vi "TEST_LoadSpec.vi"(7 "Drain!Fill":bool=TRUE, 9 "Index":i32, 10 "Level IN inches":dbl=5.0, 11 "Full Cfg in":T3={"Bench Config"={"Name"="OLR001", {"Step Levels"=0.05, "Tolerance"=0.01, "Sample Rate"=0.05, "Resistor"=100.0, "M Level Cal"=1.0, "[B Level Cal"=0.0, "Max Fill Rate"=0.002, "Empty Inches"=8.0, "Full Inches"=2.6}}, "Test Value Table "=[[98.0, 102.0, 8.5, 8.5, 8.5, 8.5, 98.0, 102.0, 8.5, 8.5, 8.5, 8.5], [98.0, 102.0, 7.91, 8.01, 7.55, 7.65, 98.0, 102.0, 7.685, 7.785, 7.325, 7.425], [197.0, 203.0, 7.46, 7.56, 7.1, 7.2, 197.0, 203.0, 7.235, 7.335, 6.875, 6.975], [296.0, 304.0, 7.01, 7.11, 6.65, 6.75, 296.0, 304.0, 6.785, 6.885, 6.425, 6.525], [395.0, 405.0, 6.56, 6.66, 6.2, 6.3, 395.0, 405.0, 6.335, 6.435, 5.975, 6.075], [494.0, 506.0, 6.11, 6.21, 5.75, 5.85, 494.0, 506.0, 5.885, 5.985, 5.525, 5.625], [593.0, 607.0, 5.66, 5.76, 5.3, 5.4, 593.0, 607.0, 5.435, 5.535, 5.075, 5.175], [692.0, 708.0, 5.21, 5.31, 4.85, 4.95, 692.0, 708.0, 4.985, 5.085, 4.625, 4.725], [791.0, 809.0, 4.76, 4.86, 4.4, 4.5, 791.0, 809.0, 4.535, 4.635, 4.175, 4.275], [890.0, 910.0, 4.31, 4.41, 3.95, 4.05, 890.0, 910.0, 4.085, 4.185, 3.725, 3.825], [989.0, 1011.0, 3.86, 3.96, 3.5, 3.6, 989.0, 1011.0, 3.635, 3.735, 3.275, 3.375], [1088.0, 1112.0, 3.41, 3.51, 3.05, 3.15, 1088.0, 1112.0, 3.185, 3.285, 2.825, 2.925], [1088.0, 1112.0, 2.5, 2.5, 2.5, 2.5, 1088.0, 1112.0, 2.5, 2.5, 2.5, 2.5]], "Table Col Titles"=[["Aohm Lo", "Aohm Hi", "A Fill Lo", "A Fill Hi", "A Drain Lo", "A Drain Hi", "Bohm Lo", "Bohm Hi", "B Fill Lo", "B Fill Hi", "B Drain Lo", "B Drain Hi"]], "cluster"={"Fill "=refnum, "Drain"=refnum, "Level PV"=refnum, "Pump Speed"=refnum, "Run Test"=refnum, "Sim"=refnum, "Jog"=refnum, "Level SP"=refnum}, "Bench Status"={"Pump Status"=refnum, "Instrumnet\n Status"=refnum}}) -> (2 "Set Point":dbl=8.5, 3 "Array":T1[](array[typedef])=[{"Specs"=[8.5, 8.5, 0.0, 102.0, 98.0, 0.0, 0.0], "LUT Status"={"ChA/!ChB"=TRUE, "Drain/!Fill"=FALSE, "In Range?"=FALSE, "Switch Range?"=FALSE, "Measure R?"=FALSE, "Vaild R?"=FALSE, "Index(n)"=0, "Index(n)-1"=0, "Index Max"=13, "Index(n-1)"=-1}}, {"Specs"=[0.0, 0.0, 0.0, 0.0, 0.0, 0.0, 0.0], "LUT Status"={"ChA/!ChB"=FALSE, "Drain/!Fill"=FALSE, "In Range?"=FALSE, "Switch Range?"=FALSE, "Measure R?"=FALSE, "Vaild R?"=FALSE, "Index(n)"=-1, "Index(n)-1"=0, "Index Max"=13, "Index(n-1)"=-2}}])   [LabVIEW 2024]
uses:
  Control Definitions/Def FullCfg.ctl
  Control Definitions/Def BenchCfg.ctl
  Control Definitions/Def PumpCtlRefs.ctl
  Control Definitions/Def_PumpSpeed.ctl
  Control Definitions/Def Bench Status.ctl
  Control Definitions/Def Spec RNG.ctl
  Control Definitions/Ded LUT_Status.ctl
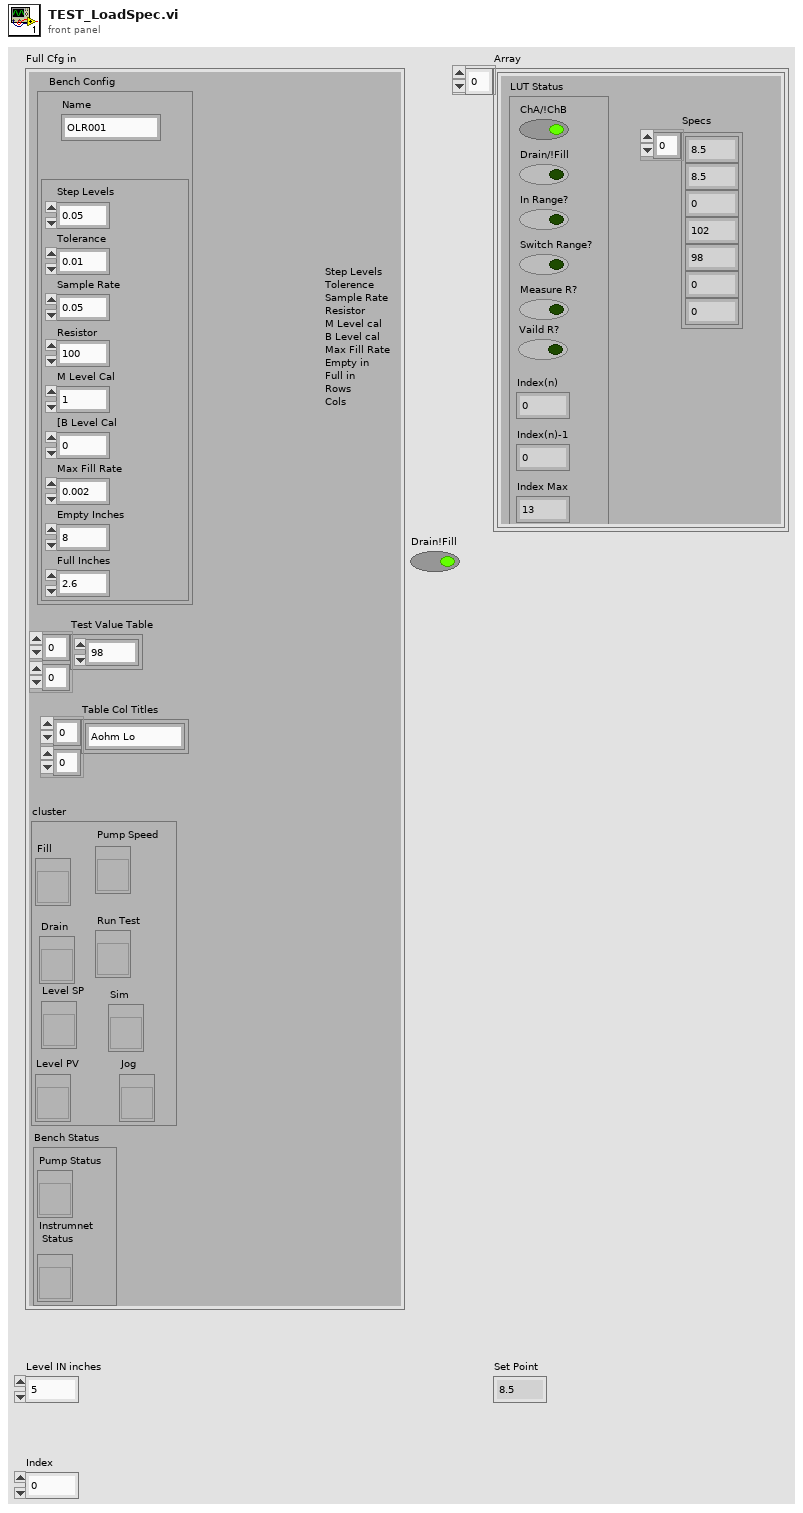
[diagram p1: front panel]
types:
  T1 = typedef "Def Spec RNG.ctl" = cluster{"Specs":dbl[], "LUT Status":T2}
  T2 = typedef "Ded LUT_Status.ctl" = cluster{"ChA/!ChB":bool, "Drain/!Fill":bool, "In Range?":bool, "Switch Range?":bool, "Measure R?":bool, "Vaild R?":bool, "Index(n)":i32, "Index(n)-1":i32, "Index Max":i32, "Index(n-1)":i32}
  T3 = typedef "Def FullCfg.ctl" = cluster{"Bench Config":T4, "Test Value Table ":dbl[][], "Table Col Titles":string[][], "cluster":T5, "Bench Status":T6}
  T4 = typedef "Def BenchCfg.ctl" = cluster{"Name":string, cluster{"Step Levels":dbl, "Tolerance":dbl, "Sample Rate":dbl, "Resistor":dbl, "M Level Cal":dbl, "[B Level Cal":dbl, "Max Fill Rate":dbl, "Empty Inches":dbl, "Full Inches":dbl}}
  T5 = typedef "Def PumpCtlRefs.ctl" = cluster{"Fill ":refnum<vi>, "Drain":refnum<vi>, "Level PV":refnum<vi>, "Pump Speed":refnum<vi>, "Run Test":refnum<vi>, "Sim":refnum<vi>, "Jog":refnum<vi>, "Level SP":refnum<vi>}
  T6 = typedef "Def Bench Status.ctl" = cluster{"Pump Status":refnum<vi>, "Instrumnet\n Status":refnum<vi>}
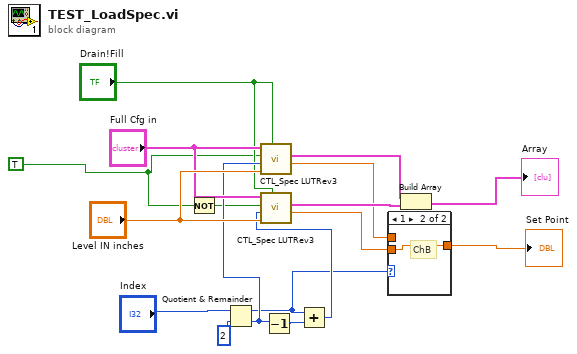
[diagram p0: block diagram]
diagram:
  w1 = TRUE ("Cha!Chb")
  n1 = Not(x=w1) -> (.not. x?=w2:bool)
  n2 = Quotient & Remainder(x="Index", y=2) -> (x-y*floor(x/y)=w4:i32, floor(x/y)=w12:i32)
  n3 = call "CTL_Spec LUTRev3.vi"("Drain!Fill"="Drain!Fill", "Level IN inches"="Level IN inches", "Index"=w12, "ChA/!ChB"=w1, "Full Cfg"="Full Cfg in") -> ("Set Point"=w5:dbl, "Spec Range Out"=w8:T1)  [unwired: 3 in, 2 out]
  n4 = Decrement(x=w12) -> (x-1=w11:i32)
  n5 = Add(x=w4, y=w11) -> (x+y=w13:i32)
  n6 = call "CTL_Spec LUTRev3.vi"("Drain!Fill"="Drain!Fill", "Level IN inches"="Level IN inches", "Index"=w13, "ChA/!ChB"=w2, "Full Cfg"="Full Cfg in") -> ("Set Point"=w7:dbl, "Spec Range Out"=w9:T1)  [unwired: 3 in, 2 out]
  n7 = case shown="1" w4 {
    tunnel: w5 -> [w18 _]
    tunnel: [w18 w19] -> w17
    tunnel: w7 -> [_ w19]
    frame 0, Default {
      # "ChA"
    }
    frame 1 {
      # "ChB"
    }
  }
  "Set Point" <- w17
  n8 = Build Array(w8, w9) -> (→"Array":T1[])
